vi "Disable PWM.vi"(7 "node-ID":u8, 8 "error in (no error)":errorcluster, 11 "interface object in":refnum<k20>) -> (0 "error out":errorcluster, 3 "interface object out":refnum<k20>)   [LabVIEW 2016]
uses:
  <vilib>/CANopenLib/CANOPEN.llb/CANopen RPDO Create.vi
  <vilib>/CANopenLib/CANOPEN.llb/CANopen RPDO Close.vi
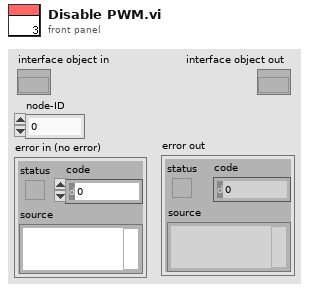
[diagram p1: front panel]
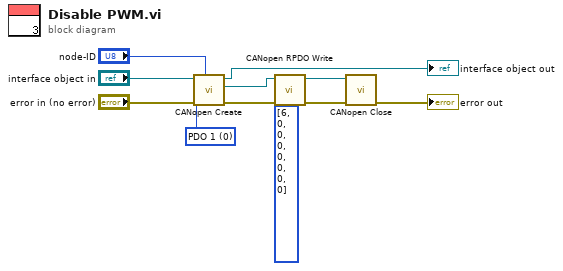
[diagram p0: block diagram]
diagram:
  w8 = u8 0 items=["PDO 1", "PDO 2", "PDO 3", "PDO 4"] ("PDO channel")
  n1 = call-poly <vilib>:"CANopen Create.vi"("node-ID"="node-ID", "error in (no error)"="error in (no error)", "PDO channel"=w8, "interface object in"="interface object in") -> ("error out"=w10:errorcluster, "RPDO object out"=w11:refnum<k20>, "interface object out"=→"interface object out":refnum<k20>)  [unwired: 5 in]
  n2 = call <vilib>:"CANopen RPDO Write.vi"("error in (no error)"=w10, "data"=u8[] [6, 0, 0, 0, 0, 0, 0, 0], "RPDO object in"=w11) -> ("error out"=w4:errorcluster, "RPDO object out"=w5:refnum<k20>)  [unwired: 7 in]
  n3 = call-poly <vilib>:"CANopen Close.vi"("error in (no error)"=w4, "RPDO object in"=w5) -> ("error out"=→"error out":errorcluster)  [unwired: 9 in]
